vi "ziExample-Module-Spectrum.vi"() -> ()   [LabVIEW 2009]
doc: "Control a Zurich instrument device via the LabOne Labview API. \nRequirements: Zurich Instruments MFLI, HF2 or UHFLI \nThis example shows how to start a spectrum modul and retrieve the Data.\n\n© Zurich Instruments AG, www.zhinst.com"
uses:
  <instrlib>/Zurich Instruments LabOne/Public/Modules/ziTypeModSpectrumWave.ctl
  <instrlib>/Zurich Instruments LabOne/Public/Modules/ziTypeModResults.ctl
  <instrlib>/Zurich Instruments LabOne/Public/Data/ziTypePollType.ctl
  <instrlib>/Zurich Instruments LabOne/Public/Modules/ziTypeModSWTriggerHeader.ctl
  <instrlib>/Zurich Instruments LabOne/Public/Modules/ziTypeModSweeperHeader.ctl
  <instrlib>/Zurich Instruments LabOne/Public/Modules/ziModSetValueDouble.vi
  <instrlib>/Zurich Instruments LabOne/Public/Modules/ziModSetValueBinary.vi
  <instrlib>/Zurich Instruments LabOne/Public/Modules/ziModSetValueDoubleArray.vi
  <instrlib>/Zurich Instruments LabOne/Zurich Instruments LabOne.lvlib
panel:
  in  "Power":bool
  in  "Window":u16(ring) items=["Rectangular", "Hann", "Hamming", "Blackman Harris"]
  in  "Absolute":bool
  in  "Spectral Density":bool
  in  "Filter Compensation":bool
  out "Error Out":errorcluster
  in  "Address":string="DEV"
  out "concatenated string":string
  out "Selected Device":string
  in  "subscribepath":string="demods/0/sample" caption="Subscribe Path"
  out "ziModResults":T1
  out "SpectrumData":cluster{"grid":dbl[], "r_avg":dbl[]}(graph)
  out "SpectrumWaveArray":T5[](array[typedef]) {"overlap" format="%f"; "nenbw" format="%f"; "center" format="%f"; "resolution" format="%f"; "aliasingReject" format="%f"; "rate" format="%f"; "bandwidth" format="%f"; "window" format="%f"; "flags" format="%f"; "sampleFormat" format="%f"; "spectrumMode" format="%f"; "sampleCount" format="%f"; "timestamp" format="%f"}
  # "ziExample-SpectrumModul.vi\nRequirements: HF2LI, UHFLI or MFLI\nsee block diagram for VI description"
  # "Tested Devices:\n- HF2LI\n- UHFLI\n- MFLI"
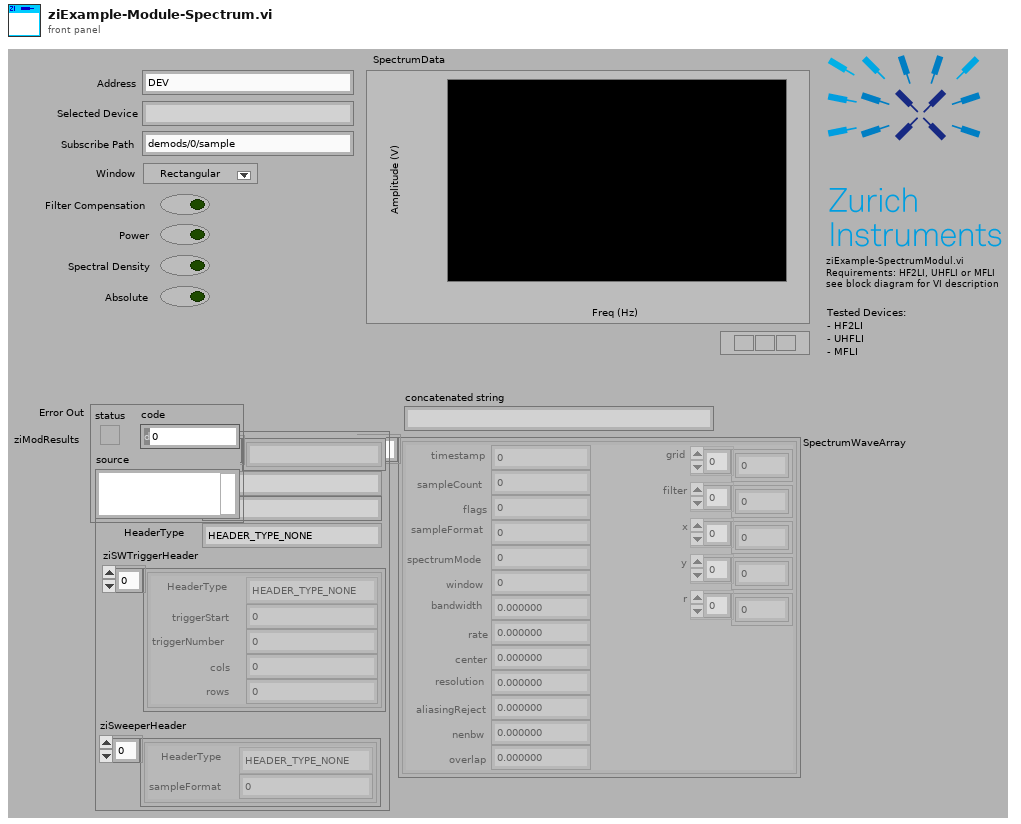
[diagram p1: front panel]
types:
  T1 = typedef "Zurich Instruments LabOne.lvlib/ziTypeModResults.ctl" = cluster{"PathArray":string[], "ValueType":T2, "NoOfResults":u64, "HeaderType":enum16{"HEADER_TYPE_NONE", "HEADER_TYPE_SWTRIGGER", "HEADER_TYPE_SWEEPER"}, "ziSWTriggerHeader":T3[], "ziSweeperHeader":T4[]}
  T2 = typedef "Zurich Instruments LabOne.lvlib/ziTypePollType.ctl" = enum16{"NONE", "DOUBLE_DATA", "INTEGER_DATA", "DEMOD_SAMPLE", "SCOPE_WAVE_HF2", "AUXIN_SAMPLE", "DIO_SAMPLE", "BYTE_ARRAY", "PWA_WAVE", "9", "10", "11", "12", "13", "14", "15", "TREE_CHANGE_DEPRI", "17", "ERROR", "19", "20", "21", "22", "23", "24", "25", "26", "27", "28", "29", "30", "31", "DOUBLE_DATA_TS", "INTEGER_DATA_TS", "34", "SCOPE_WAVE", "36", "37", "BYTE_ARRAY_TS", "39", "40", "41", "42", "43", "44", "45", "CNT_DATA", "47", "TREE_CHANGE", "49", "50", "51", "52", "53", "54", "55", "56", "57", "58", "59", "60", "61", "62", "63", "SWEEPER_DATA", "SPECTRUM_DATA", "ADVISOR_DATA", "67", "IMP_DATA"}
  T3 = typedef "Zurich Instruments LabOne.lvlib/ziTypeModSWTriggerHeader.ctl" = cluster{"HeaderType":enum8{"HEADER_TYPE_NONE", "HEADER_TYPE_SWTRIGGER", "HEADER_TYPE_SWEEPER"}, "triggerStart":u64, "triggerNumber":u64, "cols":u32, "rows":u32}
  T4 = typedef "Zurich Instruments LabOne.lvlib/ziTypeModSweeperHeader.ctl" = cluster{"HeaderType":enum8{"HEADER_TYPE_NONE", "HEADER_TYPE_SWTRIGGER", "HEADER_TYPE_SWEEPER"}, "sampleFormat":u8}
  T5 = typedef "Zurich Instruments LabOne.lvlib/ziTypeModSpectrumWave.ctl" = cluster{"timestamp":u64, "sampleCount":u64, "flags":u8, "sampleFormat":u8, "spectrumMode":u8, "window":u8, "bandwidth":dbl, "rate":dbl, "center":dbl, "resolution":dbl, "aliasingReject":dbl, "nenbw":dbl, "overlap":dbl, "grid":dbl[], "filter":dbl[], "x":dbl[], "y":dbl[], "r":dbl[]}
  T6 = typedef "Zurich Instruments LabOne.lvlib/ziTypeHandle.ctl" = cluster{"handleValid":bool, "Conn":u64, "Path Prefix":string, "Handle":u64, "Connected":bool, "Clockbase(s)":dbl}
  T7 = typedef "Zurich Instruments LabOne.lvlib/ziTypeModHandle.ctl" = cluster{"handleValid":bool, "Conn":u64, "ModHandle":u64, "moduleID":string, "Path Prefix":string}
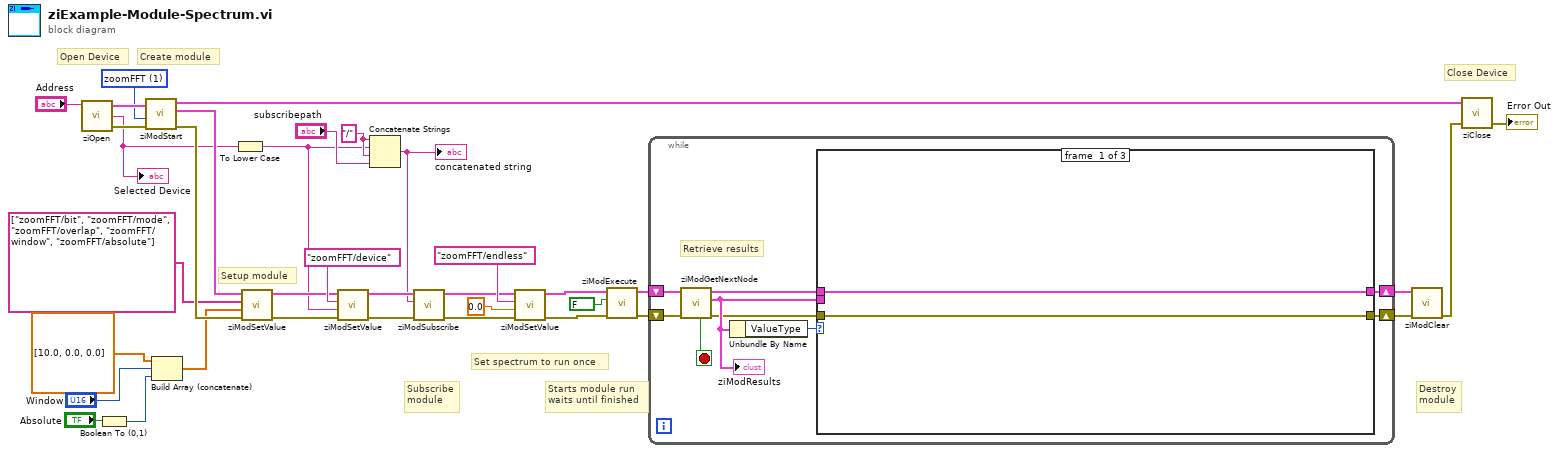
[diagram p0: block diagram]
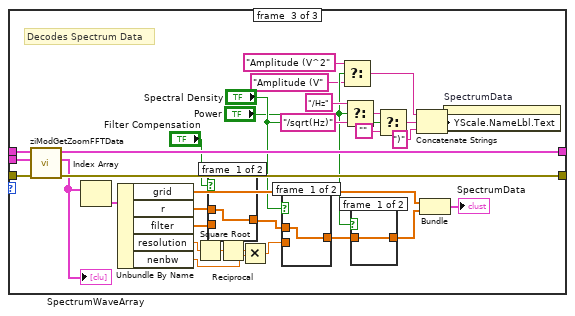
[diagram p3: hidden frame]
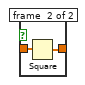
[diagram p4: hidden frame]
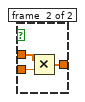
[diagram p5: hidden frame]
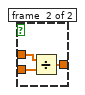
[diagram p6: hidden frame]
diagram:
  w26 = u16 1 items=["sweep", "zoomFFT", "deviceSettings", "record", "pllAdvisor", "pidAdvisor"] ("moduleID")
  w14 = "/" ("string")
  # "Close Device"
  # "Destroy\nmodule"
  # "Starts module run\nwaits until finished"
  # "Set spectrum to run once"
  # "Subscribe\nmodule"
  # "Setup module"
  # "Create module"
  # "Open Device"
  n1 = call <instrlib>:"ziOpen.vi"("Address"="Address") -> ("Error Out"=w35:errorcluster, "Selected Device"=w12:string, "HandleOut"=w36:T6)  [unwired: 3 in]
  "Selected Device" <- w12
  n2 = Boolean To (0,1)(Boolean="Absolute") -> (0, 1=w2:i16)
  n3 = call <instrlib>:"ziModStart.vi"("Error In"=w35, "module Id"=w26, "Handle In"=w36) -> ("Error Out"=w23:errorcluster, "ModHandle Out"=w22:T7, "Handle Out"=w25:T6)  [unwired: 6 in]
  n4 = Build Array (concatenate)(dbl[] [10.0, 0.0, 0.0], "Window", w2) -> (w3:dbl[])
  n5 = To Lower Case(string=w12) -> (all lower case string=w11:string)
  n6 = call-poly <instrlib>:"ziModSetValue.vi"("Error In"=w23, "Values"=w3, "Paths"=string[] ["zoomFFT/bit", "zoomFFT/mode", "zoomFFT/overlap", "zoomFFT/window", "zoomFFT/absolute"], "ModHandle In"=w22) -> ("Error Out"=w17:errorcluster, "ModHandle Out"=w20:T7)  [unwired: 6 in]
  n7 = call-poly <instrlib>:"ziModSetValue.vi"("Error In"=w17, "Data"=w11, "Path"="zoomFFT/device" ("path"), "ModHandle In"=w20) -> ("Error Out"=w18:errorcluster, "ModHandle Out"=w19:T7)  [unwired: 6 in]
  n8 = Concatenate Strings(w14, w11, w14, "subscribepath") -> (w13:string)
  "concatenated string" <- w13
  n9 = call <instrlib>:"ziModSubscribe.vi"("Error In"=w18, "Path"=w13, "ModHandle In"=w19) -> ("Error Out"=w32:errorcluster, "ModHandle Out"=w33:T7)  [unwired: 6 in]
  n10 = call-poly <instrlib>:"ziModSetValue.vi"("Error In"=w32, "Value"=0.0, "Path"="zoomFFT/endless", "ModHandle In"=w33) -> ("Error Out"=w31:errorcluster, "ModHandle Out"=w30:T7)  [unwired: 6 in]
  n11 = call <instrlib>:"ziModExecute.vi"("Error In"=w31, "Modal (F)"=FALSE ("Modal"), "ziModHandle In"=w30) -> ("Error Out"=w27:errorcluster, "ziModHandle Out"=w29:T7)  [unwired: 5 in, 1 out]
  n12 = while {
    shift-right: [w42] -> w8
    shift-left: w29 -> [w44]
    shift-right: [w41] -> w7
    shift-left: w27 -> [w45]
    stop <- w38 stop-if-true
    # "Retrieve results"
    n13 = call <instrlib>:"ziModGetNextNode.vi"("Error In"=w45, "ModHandle In"=w44) -> ("Error Out"=w39:errorcluster, "ModResults"=w40:T1, "ModHandle Out"=w43:T7, "NoData"=w38:bool)  [unwired: 6 in]
    "ziModResults" <- w40
    n14 = Unbundle By Name(w40) -> ("ValueType"=w37:T2)
    n15 = case shown="Default" w37 {
      tunnel: w43 -> [w47 w49 w80]
      tunnel: w40 -> [_ _ w81]
      tunnel: w39 -> [w46 w48 w79]
      tunnel: [w46 w48 w78] -> w41
      tunnel: [w47 w49 w77] -> w42
      frame #0 {
      }
      frame #1 {
      }
      frame #2 {
        # "Decodes Spectrum Data"
        n16 = call <instrlib>:"ziModGetZoomFFTData.vi"("Error In"=w79, "ModResults"=w81, "ModHandle In"=w80) -> ("Error Out"=w78:errorcluster, "SpectrumWaveArray"=w73:T5[], "ModHandle Out"=w77:T7)  [unwired: 6 in]
        "SpectrumWaveArray" <- w73
        n17 = Index Array(array=w73) -> (element=w76:T5)  [unwired: 1 in]
        n18 = Unbundle By Name(w76) -> ("grid"=w75:dbl[], "r"=w71:dbl[], "filter"=w70:dbl[], "resolution"=w68:dbl, "nenbw"=w65:dbl)
        n19 = Square Root(x=w68) -> (sqrt(x)=w64:dbl)
        n20 = case shown="True" "Filter Compensation" {
          tunnel: w71 -> [w89 w91]
          tunnel: [w89 w92] -> w69
          tunnel: w70 -> [_ w90]
          frame #0 {
          }
          frame #1 {
            n21 = Divide(x=w91, y=w90) -> (x/y=w92:dbl[])
          }
        }
        n22 = Reciprocal(x=w64) -> (1/x=w67:dbl)
        n23 = Multiply(x=w67, y=w65) -> (x*y=w66:dbl)
        n24 = case shown="True" "Spectral Density" {
          tunnel: w69 -> [w85 w87]
          tunnel: [w85 w88] -> w63
          tunnel: w66 -> [_ w86]
          frame #0 {
          }
          frame #1 {
            n25 = Multiply(x=w87, y=w86) -> (x*y=w88:dbl[])
          }
        }
        n26 = Select(t="Amplitude (V^2", s="Power", f="Amplitude (V") -> (s? t:f=w53:string)
        n27 = Select(t="/Hz", s="Power", f="/sqrt(Hz)") -> (s? t:f=w58:string)
        n28 = case shown="True" "Power" {
          tunnel: w63 -> [w82 w84]
          tunnel: [w82 w83] -> w62
          frame #0 {
          }
          frame #1 {
            n29 = Square(x=w84) -> (x^2=w83:dbl[])
          }
        }
        n30 = Select(t=w58, s="Spectral Density", f="") -> (s? t:f=w52:string)
        n31 = Concatenate Strings(w53, w52, ")") -> (w51:string)
        n32 = Bundle("grid"=w75, "r"=w62) -> (→"SpectrumData":cluster{"grid":dbl[], "r":dbl[]})  [unwired: 1 in]
        n33 = property on="SpectrumData" class="XYGraph (strict)"("YScale.NameLbl.Text"=w51) -> ()  [unwired: 2 in, 2 out]
      }
    }
  }
  n34 = call <instrlib>:"ziModClear.vi"("Error In"=w7, "ziModHandle In"=w8) -> ("Error Out"=w24:errorcluster)  [unwired: 7 in, 1 out]
  n35 = call <instrlib>:"ziClose.vi"("Error In"=w24, "Handle In"=w25) -> ("Error Out"=→"Error Out":errorcluster)  [unwired: 2 in, 1 out]
